vi "Latch Boolean.vi"(1 "Boolean Input":bool) -> (0 "Boolean Output":bool)   [LabVIEW 2011]
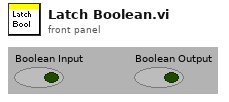
[diagram p1: front panel]
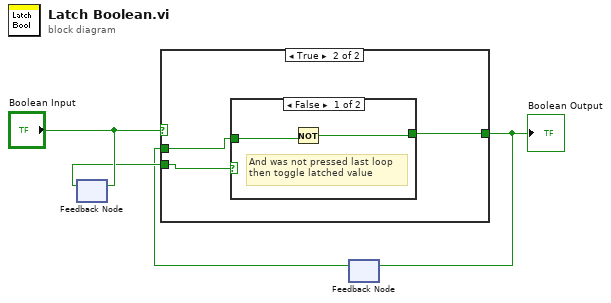
[diagram p0: block diagram]
diagram:
  n1 = feedback-in #1("Boolean Input") -> ()
  n2 = feedback #1() -> (w3:bool)  [unwired: 1 out]
  n3 = feedback #2() -> (w1:bool)  [unwired: 1 out]
  n4 = case shown="True" "Boolean Input" {
    tunnel: [w5 w8] -> w2
    tunnel: w3 -> [_ w6]
    tunnel: w1 -> [w5 w7]
    frame False {
      # "then do nothing"
      # "If button is not pressed"
    }
    frame True {
      n5 = case shown="False" w6 {
        tunnel: [w10 w11] -> w8
        tunnel: w7 -> [w9 w11]
        frame False {
          # "And was not pressed last loop\nthen toggle latched value"
          n6 = Not(x=w9) -> (.not. x?=w10:bool)
        }
        frame True {
          # "And was pressed last loop\nthen hold current latched value"
        }
      }
    }
  }
  "Boolean Output" <- w2
  n7 = feedback-in #2(w2) -> ()
